vi "Detect ISw.vi"(9 "Side Gyro Data":T3={"Time"=0.0, "Gyro Array Data"=[], "Gyro Negation"=[], "Gyro Data"={"Gyro X"=0.0, "Gyro Y"=0.0, "Gyro Z"=0.0}, "Gyro Latency"=0.0, "Normalization Time"=640.0, "Sampling Rate"=0.0}, 10 "Side Event Data":T1={"Event Data"={"LR"={"Phase"="LR", "On"=FALSE, "Last On Time"=0.0, "Duration"=0.0, "Crossing Time"=0.0, "Time since LR"=0.0, "Time Since TSw"=0.0, "Min gyro Z"=0.0, "Time since LR?"=FALSE, "Time since TSw?"=FALSE, "Min gyro Z?"=FALSE, "Crossing?"=FALSE}, "MSt"={"Phase"="MSt", "On"=FALSE, "Last On Time"=0.0, "Duration"=0.0}, "TSt"={"Phase"="TSt", "On"=FALSE, "Last On Time"=0.0, "Duration"=0.0}, "PSw"={"Phase"="PSw", "On"=FALSE, "Last On Time"=0.0, "Duration"=0.0}, "ISw"={"Phase"="ISw", "On"=FALSE, "Last On Time"=0.0, "Duration"=0.0, "Peak Time"=0.0, "Time since LR"=0.0, "Time since ISw"=0.0, "Time since LR?"=FALSE, "Time since ISw?"=FALSE, "Peak?"=FALSE}, "MSw"={"Phase"="MSw", "On"=FALSE, "Last On Time"=0.0, "Duration"=0.0, "Crossing time"=0.0, "Time since LR"=0.0, "Time since MSw"=0.0, "Time since ISw"=0.0, "Time since LR?"=FALSE, "Time since MSw?"=FALSE, "Time since ISw?"=FALSE, "Crossing?"=FALSE}, "TSw"={"Phase"="TSw", "On"=FALSE, "Last On Time"=0.0, "Duration"=0.0, "Peak time"=0.0, "Time since LR"=0.0, "Time since TSw"=0.0, "Time since LR?"=FALSE, "Time since TSw?"=FALSE, "Peak?"=FALSE}}, "Mean Cycle Duration"=0.0, "Event Detected?"=FALSE, "Last Event Detected"=0, "Num Cycles"=0.0, "GPD Log"=refnum, "Last Event Time"=0.0}, 11 "GPD Parameters":T2={"% Cycle Delay"=0.0, "Min % Cycle LR to ISw "=0.0, "Min % Cycle LR to MSw"=0.0, "Min % Cycle LR to TSw"=0.0, "Max % Cycle ISw to MSw"=0.0, "Min % Cycle TSw to LR"=0.0, "Max % Cycle TSw to LR"=0.0, "LR Min Gyro Z Threshold"=0.0, "LR Min Gyro Z Width"=0.0, "ISw Peak Threshold"=0.0, "ISw Peak Width"=0.0, "TSw Valley Threshold"=0.0, "TSw Valley Width (ms)"=7.0, "Max Cycle Time (s)"=0.0, "Mean Computation Window"=0.0, "CP subject?"=FALSE}) -> (1 "Side Gyro Data":T3={"Time"=0.0, "Gyro Array Data"=[], "Gyro Negation"=[], "Gyro Data"={"Gyro X"=0.0, "Gyro Y"=0.0, "Gyro Z"=0.0}, "Gyro Latency"=0.0, "Normalization Time"=640.0, "Sampling Rate"=0.0}, 2 "Side Event Data":T1={"Event Data"={"LR"={"Phase"="LR", "On"=FALSE, "Last On Time"=0.0, "Duration"=0.0, "Crossing Time"=0.0, "Time since LR"=0.0, "Time Since TSw"=0.0, "Min gyro Z"=0.0, "Time since LR?"=FALSE, "Time since TSw?"=FALSE, "Min gyro Z?"=FALSE, "Crossing?"=FALSE}, "MSt"={"Phase"="MSt", "On"=FALSE, "Last On Time"=0.0, "Duration"=0.0}, "TSt"={"Phase"="TSt", "On"=FALSE, "Last On Time"=0.0, "Duration"=0.0}, "PSw"={"Phase"="PSw", "On"=FALSE, "Last On Time"=0.0, "Duration"=0.0}, "ISw"={"Phase"="ISw", "On"=FALSE, "Last On Time"=0.0, "Duration"=0.0, "Peak Time"=0.0, "Time since LR"=0.0, "Time since ISw"=0.0, "Time since LR?"=FALSE, "Time since ISw?"=FALSE, "Peak?"=FALSE}, "MSw"={"Phase"="MSw", "On"=FALSE, "Last On Time"=0.0, "Duration"=0.0, "Crossing time"=0.0, "Time since LR"=0.0, "Time since MSw"=0.0, "Time since ISw"=0.0, "Time since LR?"=FALSE, "Time since MSw?"=FALSE, "Time since ISw?"=FALSE, "Crossing?"=FALSE}, "TSw"={"Phase"="TSw", "On"=FALSE, "Last On Time"=0.0, "Duration"=0.0, "Peak time"=0.0, "Time since LR"=0.0, "Time since TSw"=0.0, "Time since LR?"=FALSE, "Time since TSw?"=FALSE, "Peak?"=FALSE}}, "Mean Cycle Duration"=0.0, "Event Detected?"=FALSE, "Last Event Detected"=0, "Num Cycles"=0.0, "GPD Log"=refnum, "Last Event Time"=0.0}, 3 "GPD Parameters":T2={"% Cycle Delay"=0.0, "Min % Cycle LR to ISw "=0.0, "Min % Cycle LR to MSw"=0.0, "Min % Cycle LR to TSw"=0.0, "Max % Cycle ISw to MSw"=0.0, "Min % Cycle TSw to LR"=0.0, "Max % Cycle TSw to LR"=0.0, "LR Min Gyro Z Threshold"=0.0, "LR Min Gyro Z Width"=0.0, "ISw Peak Threshold"=0.0, "ISw Peak Width"=0.0, "TSw Valley Threshold"=0.0, "TSw Valley Width (ms)"=7.0, "Max Cycle Time (s)"=0.0, "Mean Computation Window"=0.0, "CP subject?"=FALSE}, 4 "ISW Detected?":bool)   [LabVIEW 2019]
uses:
  Controls/Gyro Side Data.ctl
  Controls/Gyro Negation.ctl
  Controls/GPD Side Parameters.ctl
  Controls/Side Event Data.ctl
  <vilib>/ptbypt/NI_PtbyPt.lvlib
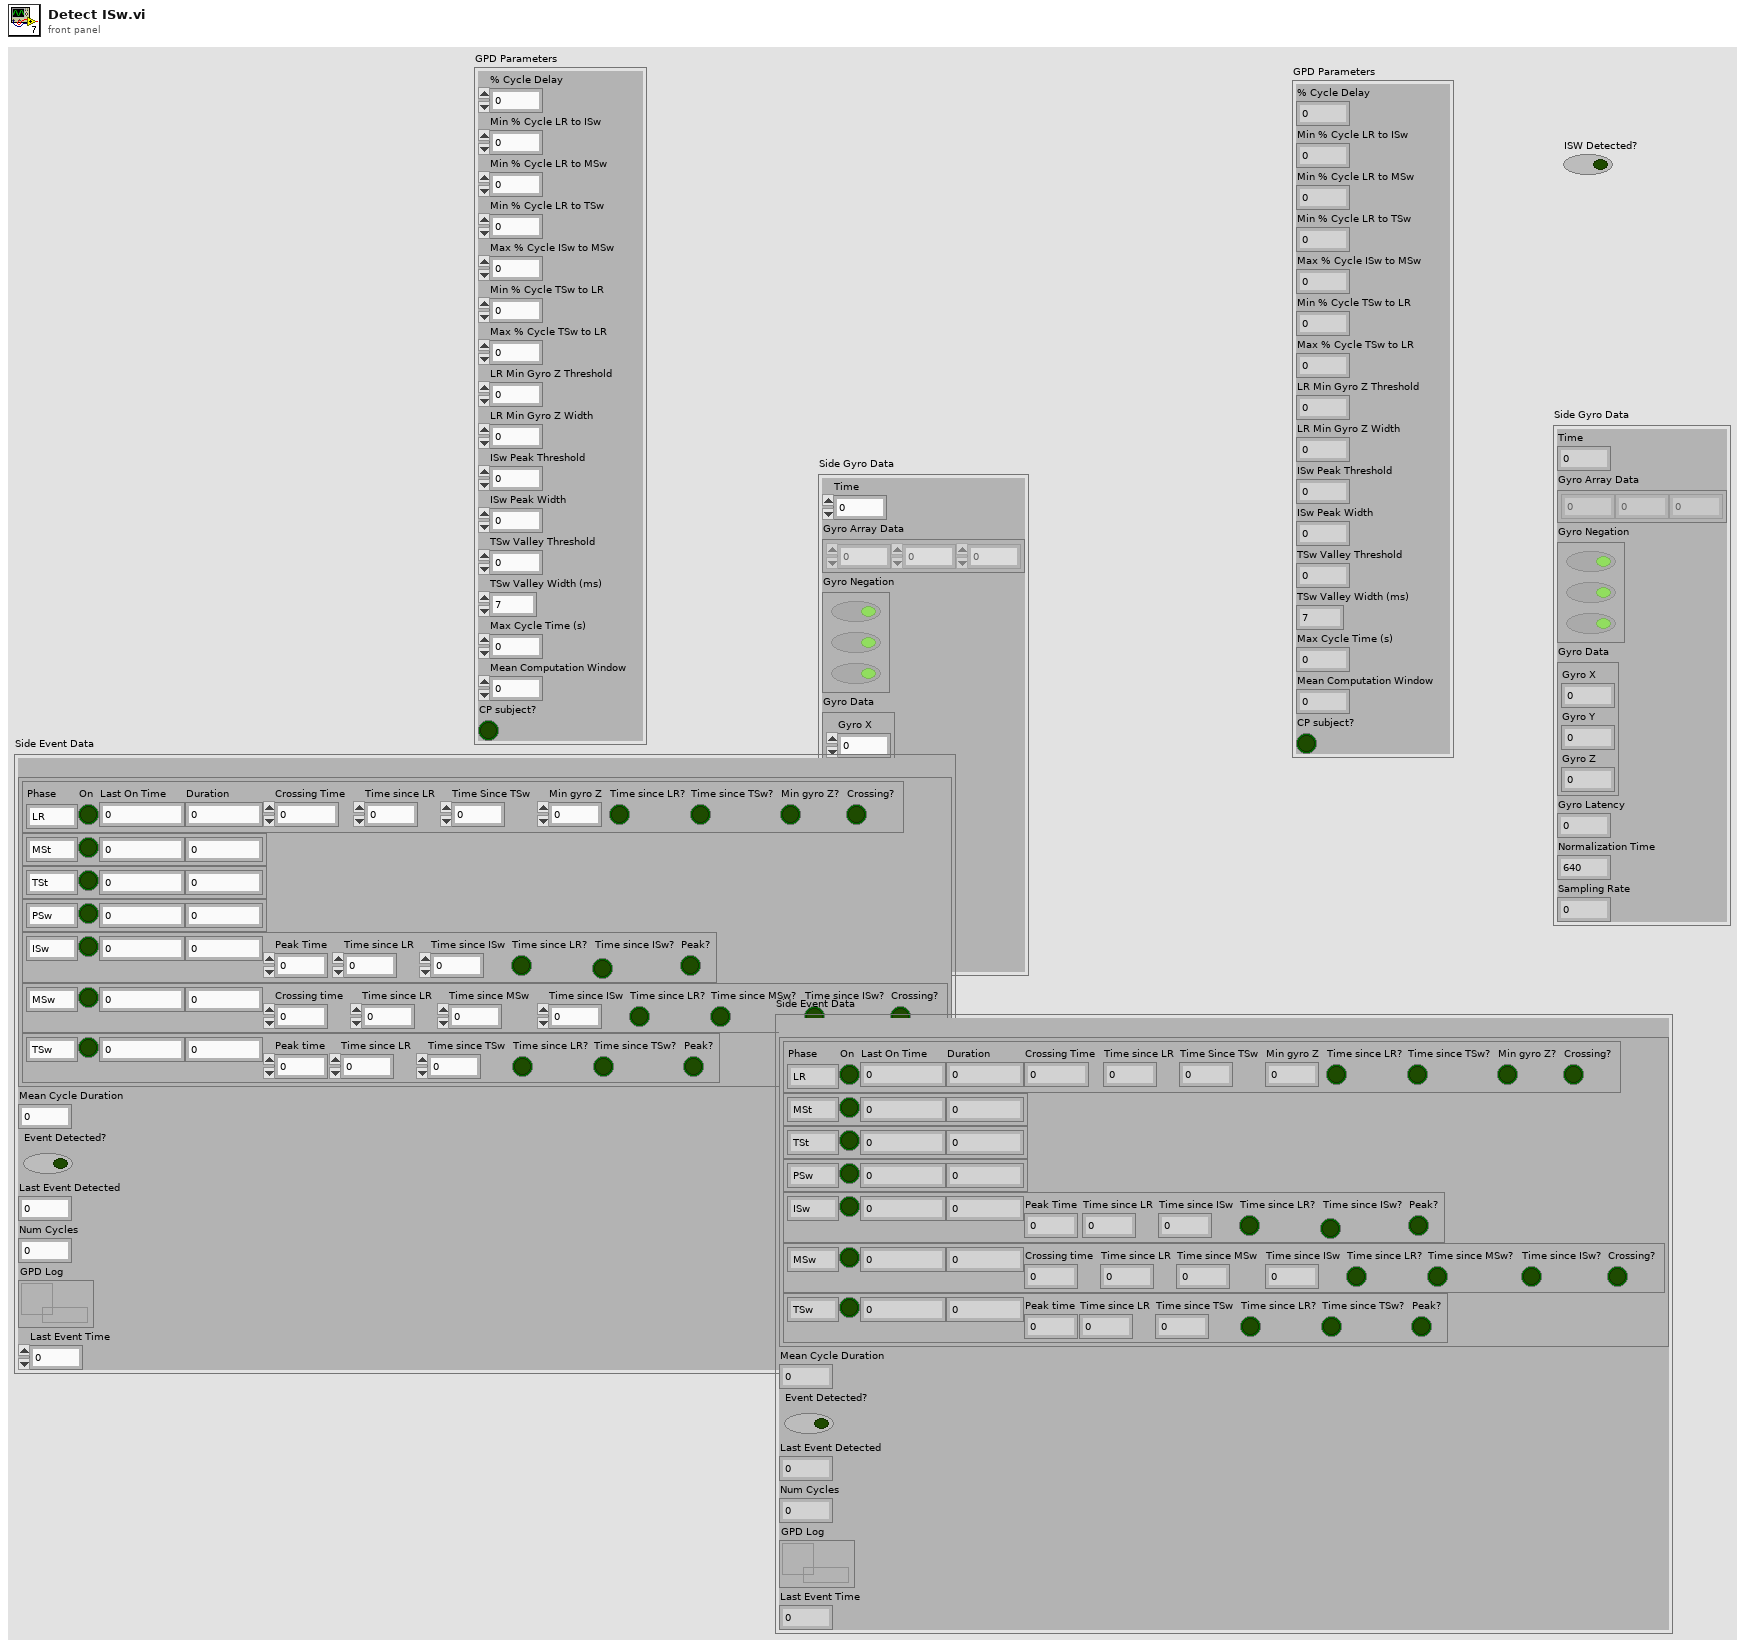
[diagram p1: front panel]
types:
  T1 = typedef "Side Event Data.ctl" = cluster{"Event Data":cluster{"LR":cluster{"Phase":string, "On":bool, "Last On Time":dbl, "Duration":dbl, "Crossing Time":dbl, "Time since LR":dbl, "Time Since TSw":dbl, "Min gyro Z":dbl, "Time since LR?":bool, "Time since TSw?":bool, "Min gyro Z?":bool, "Crossing?":bool}, "MSt":cluster{"Phase":string, "On":bool, "Last On Time":dbl, "Duration":dbl}, "TSt":cluster{"Phase":string, "On":bool, "Last On Time":dbl, "Duration":dbl}, "PSw":cluster{"Phase":string, "On":bool, "Last On Time":dbl, "Duration":dbl}, "ISw":cluster{"Phase":string, "On":bool, "Last On Time":dbl, "Duration":dbl, "Peak Time":dbl, "Time since LR":dbl, "Time since ISw":dbl, "Time since LR?":bool, "Time since ISw?":bool, "Peak?":bool}, "MSw":cluster{"Phase":string, "On":bool, "Last On Time":dbl, "Duration":dbl, "Crossing time":dbl, "Time since LR":dbl, "Time since MSw":dbl, "Time since ISw":dbl, "Time since LR?":bool, "Time since MSw?":bool, "Time since ISw?":bool, "Crossing?":bool}, "TSw":cluster{"Phase":string, "On":bool, "Last On Time":dbl, "Duration":dbl, "Peak time":dbl, "Time since LR":dbl, "Time since TSw":dbl, "Time since LR?":bool, "Time since TSw?":bool, "Peak?":bool}}, "Mean Cycle Duration":dbl, "Event Detected?":bool, "Last Event Detected":i32, "Num Cycles":dbl, "GPD Log":refnum<queue>, "Last Event Time":dbl}
  T2 = typedef "GPD Side Parameters.ctl" = cluster{"% Cycle Delay":dbl, "Min % Cycle LR to ISw ":dbl, "Min % Cycle LR to MSw":dbl, "Min % Cycle LR to TSw":dbl, "Max % Cycle ISw to MSw":dbl, "Min % Cycle TSw to LR":dbl, "Max % Cycle TSw to LR":dbl, "LR Min Gyro Z Threshold":dbl, "LR Min Gyro Z Width":dbl, "ISw Peak Threshold":dbl, "ISw Peak Width":dbl, "TSw Valley Threshold":dbl, "TSw Valley Width (ms)":dbl, "Max Cycle Time (s)":dbl, "Mean Computation Window":dbl, "CP subject?":bool}
  T3 = typedef "Gyro Side Data.ctl" = cluster{"Time":dbl, "Gyro Array Data":dbl[], "Gyro Negation":T4, "Gyro Data":cluster{"Gyro X":dbl, "Gyro Y":dbl, "Gyro Z":dbl}, "Gyro Latency":dbl, "Normalization Time":dbl, "Sampling Rate":dbl}
  T4 = typedef "Gyro Negation.ctl" = bool[]
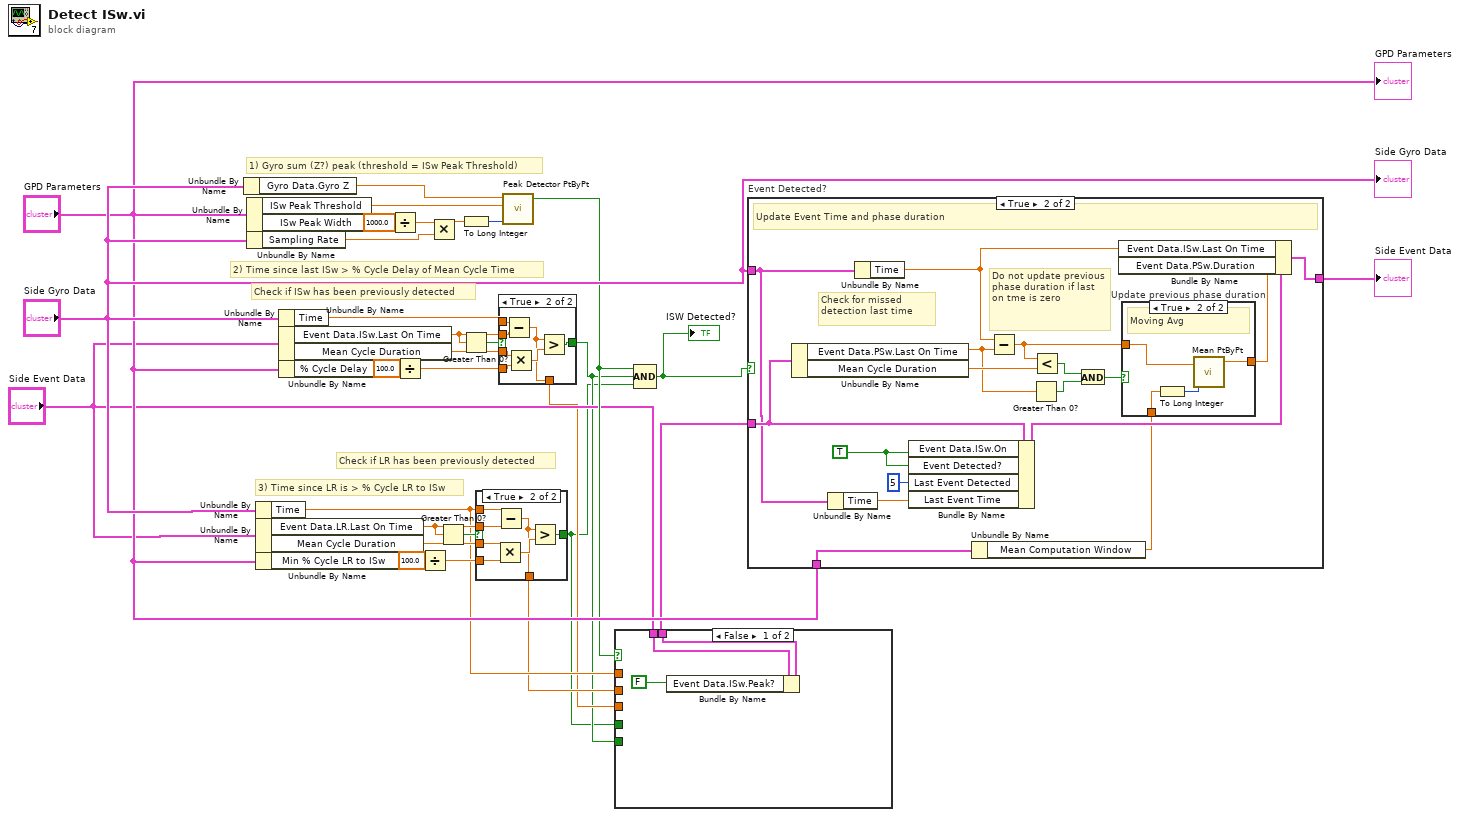
[diagram p0: block diagram]
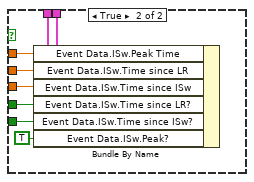
[diagram p2: hidden frame]
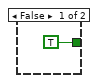
[diagram p3: hidden frame]
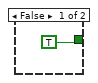
[diagram p4: hidden frame]
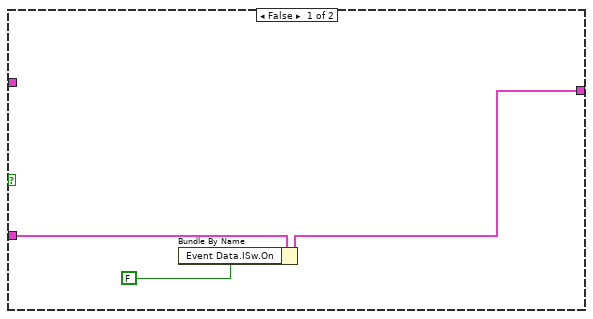
[diagram p5: hidden frame]
diagram:
  # "Check if LR has been previously detected"
  # "3) Time since LR is > % Cycle LR to ISw"
  # "2) Time since last ISw > % Cycle Delay of Mean Cycle Time"
  # "Check if ISw has been previously detected"
  # "1) Gyro sum (Z?) peak (threshold = ISw Peak Threshold)"
  n1 = Unbundle By Name("Side Gyro Data") -> ("Gyro Data.Gyro Z"=w9:dbl)
  n2 = Unbundle By Name("GPD Parameters") -> ("ISw Peak Threshold"=w32:dbl, "ISw Peak Width"=w30:dbl)
  n3 = Unbundle By Name("Side Gyro Data") -> ("Sampling Rate"=w29:dbl)
  n4 = Unbundle By Name("Side Gyro Data") -> ("Time"=w5:dbl)
  n5 = Unbundle By Name("Side Event Data") -> ("Event Data.LR.Last On Time"=w10:dbl, "Mean Cycle Duration"=w14:dbl)
  n6 = Unbundle By Name("GPD Parameters") -> ("Min % Cycle LR to ISw"=w12:dbl)
  n7 = Unbundle By Name("Side Gyro Data") -> ("Time"=w19:dbl)
  n8 = Unbundle By Name("Side Event Data") -> ("Event Data.ISw.Last On Time"=w23:dbl, "Mean Cycle Duration"=w20:dbl)
  n9 = Unbundle By Name("GPD Parameters") -> ("% Cycle Delay"=w18:dbl)
  n10 = Divide(x=w30, y=1000.0) -> (x/y=w28:dbl)
  n11 = Divide(x=w18, y=100.0) -> (x/y=w21:dbl)
  n12 = Divide(x=w12, y=100.0) -> (x/y=w13:dbl)
  n13 = Multiply(x=w28, y=w29) -> (x*y=w26:dbl)
  n14 = Greater Than 0?(x=w10) -> (x > 0?=w11:bool)
  n15 = To Long Integer(number=w26) -> (32bit integer=w27:i32)
  n16 = Greater Than 0?(x=w23) -> (x > 0?=w22:bool)
  n17 = case shown="True" w11 {
    tunnel: w5 -> [_ w41]
    tunnel: w10 -> [_ w40]
    tunnel: w14 -> [_ w39]
    tunnel: w13 -> [_ w37]
    tunnel: [TRUE w36] -> w1
    tunnel: [_ w35] -> w4
    frame False {
    }
    frame True {
      n18 = Multiply(x=w39, y=w37) -> (x*y=w38:dbl)
      n19 = Subtract(x=w41, y=w40) -> (x-y=w35:dbl)
      n20 = Greater?(x=w35, y=w38) -> (0:w36:bool)
    }
  }
  n21 = case shown="True" w22 {
    tunnel: w19 -> [_ w49]
    tunnel: w23 -> [_ w48]
    tunnel: w20 -> [_ w47]
    tunnel: w21 -> [_ w46]
    tunnel: [TRUE w44] -> w2
    tunnel: [_ w43] -> w3
    frame False {
    }
    frame True {
      n22 = Subtract(x=w49, y=w48) -> (x-y=w43:dbl)
      n23 = Multiply(x=w47, y=w46) -> (x*y=w45:dbl)
      n24 = Greater?(x=w43, y=w45) -> (0:w44:bool)
    }
  }
  n25 = call <vilib>:"Peak Detector PtByPt.vi"("x"=w9, "threshold peak"=w32, "width"=w27) -> ("peak"=w8:bool)  [unwired: 2 in, 2 out]
  n26 = case shown="False" w8 {
    tunnel: "Side Event Data" -> [w51 w60]
    tunnel: [w50 w59] -> w6
    tunnel: w5 -> [_ w58]
    tunnel: w4 -> [_ w57]
    tunnel: w3 -> [_ w56]
    tunnel: w2 -> [_ w54]
    tunnel: w1 -> [_ w55]
    frame False {
      n27 = Bundle By Name(cluster=w51, "Event Data.ISw.Peak?"=FALSE) -> (w50:T1)
    }
    frame True {
      n28 = Bundle By Name(cluster=w60, "Event Data.ISw.Peak Time"=w58, "Event Data.ISw.Time since LR"=w57, "Event Data.ISw.Time since ISw"=w56, "Event Data.ISw.Time since LR?"=w55, "Event Data.ISw.Time since ISw?"=w54, "Event Data.ISw.Peak?"=TRUE) -> (w59:T1)
    }
  }
  n29 = Compound Arithmetic op=AND(w8, w2, w1) -> (w16:bool)
  "ISW Detected?" <- w16
  n30 = case "Event Detected?" shown="True" w16 {
    tunnel: w6 -> [w62 w79]
    tunnel: [w61 w80] -> w33
    tunnel: "GPD Parameters" -> [_ w72]
    tunnel: "Side Gyro Data" -> [_ w64]
    frame False {
      n31 = Bundle By Name(cluster=w62, "Event Data.ISw.On"=FALSE) -> (w61:T1)
    }
    frame True {
      w75 = TRUE
      # "Do not update previous phase duration if last on tme is zero"
      # "Check for missed detection last time"
      # "Update Event Time and phase duration"
      n32 = Unbundle By Name(w79) -> ("Event Data.PSw.Last On Time"=w69:dbl, "Mean Cycle Duration"=w78:dbl)
      n33 = Unbundle By Name(w64) -> ("Time"=w65:dbl)
      n34 = Unbundle By Name(w64) -> ("Time"=w70:dbl)
      n35 = Bundle By Name(cluster=w79, "Event Data.ISw.On"=w75, "Event Detected?"=w75, "Last Event Detected"=5, "Last Event Time"=w65) -> (w73:T1)
      n36 = Unbundle By Name(w72) -> ("Mean Computation Window"=w71:dbl)
      n37 = Subtract(x=w70, y=w69) -> (x-y=w77:dbl)
      n38 = Greater Than 0?(x=w69) -> (x > 0?=w67:bool)
      n39 = Less?(x=w77, y=w78) -> (x < y?=w68:bool)
      n40 = And(x=w68, y=w67) -> (x .and. y?=w66:bool)
      n41 = case "Update previous phase duration" shown="True" w66 {
        tunnel: w77 -> [w81 w84]
        tunnel: [w81 w85] -> w76
        tunnel: w71 -> [_ w82]
        frame False {
        }
        frame True {
          # "Moving Avg"
          n42 = To Long Integer(number=w82) -> (32bit integer=w83:i32)
          n43 = call <vilib>:"Mean PtByPt.vi"("x"=w84, "sample length"=w83) -> ("mean"=w85:dbl)  [unwired: 2 in, 1 out]
        }
      }
      n44 = Bundle By Name(cluster=w73, "Event Data.ISw.Last On Time"=w70, "Event Data.PSw.Duration"=w76) -> (w80:T1)
    }
  }
  "Side Event Data" <- w33
  "Side Gyro Data" <- "Side Gyro Data"
  "GPD Parameters" <- "GPD Parameters"
